vi "FTW-TransferClient-Construct.vi"(5 "Username":string, 7 "Password":string, 9 "Headers":cluster{"Key":string, "Value":string}[](array[cluster]), 11 "error in":errorcluster) -> (4 "Transfer Client":refnum<k24>, 15 "error out":errorcluster)   [LabVIEW 2014]
panel:
  # "Inputs"
  # "Outputs"
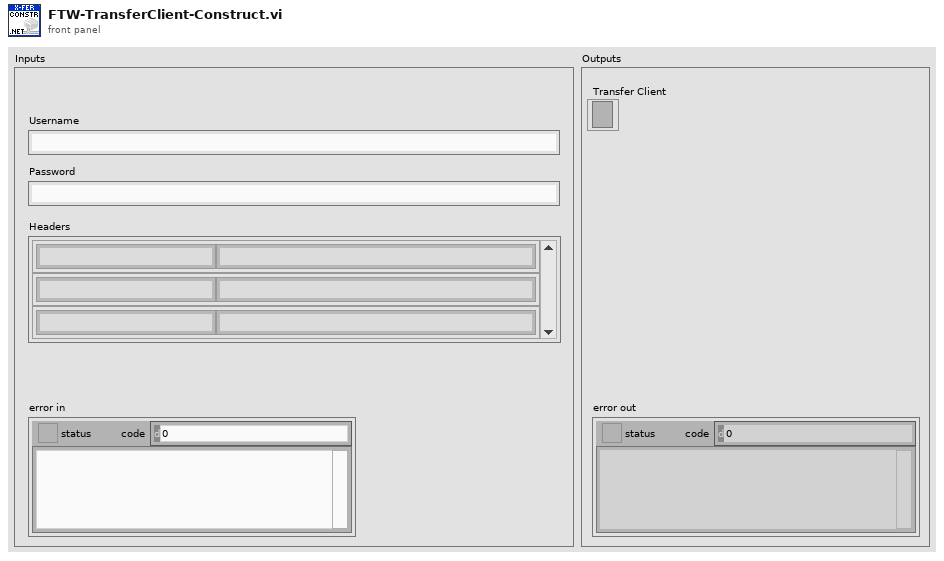
[diagram p1: front panel]
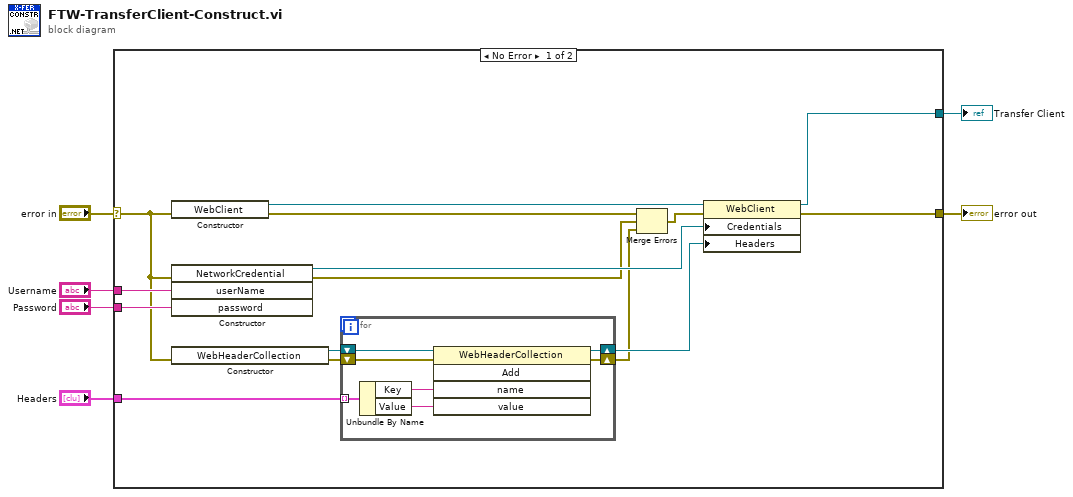
[diagram p0: block diagram]
diagram:
  n1 = case shown="No Error" "error in" {
    selector: "error in" -> [w8 w29]
    tunnel: [w11 w29] -> w5
    tunnel: [w7 _] -> w4
    tunnel: "Username" -> [w13 _]
    tunnel: "Password" -> [w12 _]
    tunnel: "Headers" -> [w9 _]
    frame No Error {
      n2 = constructor class="WebClient"(error in=w8) -> (reference out=w21:refnum<k24>, error out=w10:errorcluster)  [unwired: 2 in, 1 out]
      n3 = constructor class="NetworkCredential"(error in=w8, "userName"=w13, "password"=w12) -> (reference out=w20:refnum<k24>, error out=w16:errorcluster)  [unwired: 2 in, 3 out]
      n4 = constructor class="WebHeaderCollection"(error in=w8) -> (reference out=w19:refnum<k24>, error out=w18:errorcluster)  [unwired: 2 in, 1 out]
      n5 = for {
        shift-right: [w26] -> w17
        shift-left: w19 -> [w28]
        shift-right: [w25] -> w15
        shift-left: w18 -> [w27]
        tunnel: w9 -> [w24] mode=indexing
        n6 = Unbundle By Name(w24) -> ("Key"=w23:string, "Value"=w22:string)
        n7 = invoke class="WebHeaderCollection" method="Add"(reference=w28, error in=w27, "name"=w23, "value"=w22) -> (reference out=w26:refnum<k24>, error out=w25:errorcluster)  [unwired: 1 in, 3 out]
      }
      n8 = Merge Errors(w10, w16, w15) -> (w14:errorcluster)
      n9 = property class="WebClient"(reference=w21, error in=w14, "Credentials"=w20, "Headers"=w17) -> (reference out=w7:refnum<k24>, error out=w11:errorcluster)
    }
    frame Error {
    }
  }
  "error out" <- w5
  "Transfer Client" <- w4
